vi "YKMW100 Clear Output Buffer.vi"(0 "VISA session":refnum<visa-resource-name>="MW100", 11 "error in (no error)":errorcluster) -> (4 "dup VISA session":refnum<visa-resource-name>, 15 "error out":errorcluster)   [LabVIEW 2009]
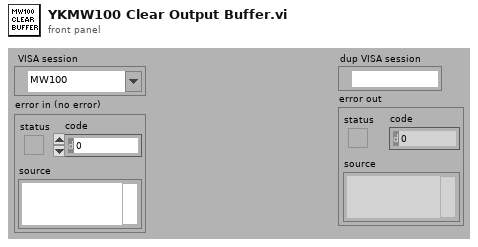
[diagram p1: front panel]
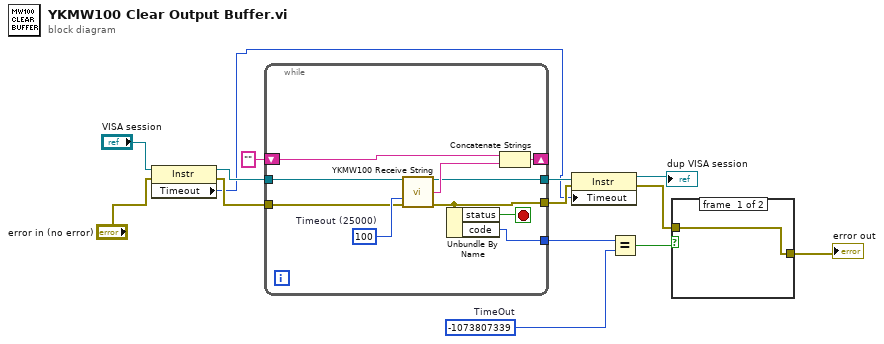
[diagram p0: block diagram]
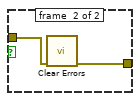
[diagram p2: hidden frame]
diagram:
  w12 = -1073807339  # TimeOut
  n1 = property class="Instr"(reference="VISA session", error in="error in (no error)") -> (reference out=w6:refnum<visa-resource-name>, error out=w7:errorcluster, "Timeout"=w1:u32)
  n2 = while {
    tunnel: w7 -> [w22]
    shift-right: [w19] -> _
    shift-left: "" -> [w20]
    tunnel: [w18] -> w5
    tunnel: [w17] -> w13
    tunnel: [w16] -> w2
    tunnel: w6 -> [w15]
    stop <- w24 stop-if-true
    w23 = u32 100  # Timeout (25000)
    n3 = call "YKMW100 Receive String.vi"("VISA session"=w15, "Timeout (25000)"=w23, "error in (no error)"=w22) -> ("dup VISA session"=w18:refnum<visa-resource-name>, "Read Buffer"=w21:string, "error out"=w16:errorcluster)  [unwired: 10 in]
    n4 = Unbundle By Name(w16) -> ("status"=w24:bool, "code"=w17:i32)
    n5 = Concatenate Strings(w20, w21) -> (w19:string)
  }
  n6 = property class="Instr"(reference=w5, error in=w2, "Timeout"=w1) -> (reference out=→"dup VISA session":refnum<visa-resource-name>, error out=w3:errorcluster)
  n7 = Equal?(x=w13, y=w12) -> (x = y?=w11:bool)
  n8 = case shown="False" w11 {
    tunnel: w3 -> [w25 w27]
    tunnel: [w25 w26] -> w10
    frame #0 {
    }
    frame #1 {
      n9 = call <vilib>:"Clear Errors.vi"("error in (no error)"=w27) -> ("error out"=w26:errorcluster)  [unwired: 6 in]
    }
  }
  "error out" <- w10
